vi "CC Script GUI.vi"(10 "Standalone":bool=TRUE, 11 "Cmd Qs":T1) -> ()   [LabVIEW 2021]
uses:
  Subsystems/SS cluster Command Queues.ctl
  Subsystems/SS typedef Cmd Queue Reference.ctl
  Subsystems/SS typedef cluster Instrument Command Queue Data.ctl
  CC cluster Script Panel Defaults.ctl
  typedefs/CC Script Step.ctl
  typedefs/CC enum Script Action.ctl
  typedefs/CC cluster Exposure.ctl
  Detector/Detector Class/Detector enum Detector Integration Mode.ctl
  typedefs/CC cluster Object.ctl
  typedefs/CC cluster sidereal rate.ctl
  typedefs/CC cluster RA and DEC.ctl
  typedefs/cc cluster muRA muDEC.ctl
  Telescope/CC cluster Telescope Offsets.ctl
  typedefs/CC cluster Acquire Parameters.ctl
  Subsystems/SS cluster Script Status Queue.ctl
  typedefs/CC cluster Random Dithering.ctl
  typedefs/CC Dithering.ctl
  typedefs/CC cluster Offset Dithering.ctl
  typedefs/CC Dithering Offsets.ctl
  typedefs/CC cluster Observation Record.ctl
  Subsystems/SS cluster New Image Data.ctl
  hk-channel-class/HK Item/HK Item.lvclass
  Subsystems/SS cluster Data Queue type.ctl
  typedefs/CC cluster Observation.ctl
  Observation Queue/CC enum Observation Status.ctl
  typedefs/CC cluster Observation Dither Options.ctl
  typedefs/CC enum Dither Selection.ctl
  typedefs/CC cluster Script.ctl
  typedefs/CC cluster Script Status Data.ctl
  typedefs/CC cluster Pause Parameters.ctl
  Filter Wheel/FW cmd Q Move Parameters.ctl
  Logging/CC enum Current Values Action.ctl
  Focus/Focus cluster MoveFocus Command Parameters.ctl
  CC Rd Wr Script Action.ctl
  e34a80dd-ae96-40f3-85ec-da568b1fc0c6.vi
  fb980131-14b8-4ba4-a5ba-d8795c8df878.vi
  73e8f019-b90d-454d-a375-f578a22e9470.vi
  6180e3d0-9506-4a5f-afbf-da5a1e2ce68c.vi
  79eba822-2b6b-4a1a-8f0f-f154aabb2b36.vi
  hk-channel-class/HK Table/HK Table.lvclass
  <vilib>/Utility/Data Type/NI_Data Type.lvlib
panel:
  in  "Script Path":path
  in  "Pause Button":bool
  out "Running":bool
  in  "Close":bool
  in  "Stop Script":bool
  in  "New Script":bool
  in  "Edit Script":bool
  in  "Run Script":bool
  in  "Script":string(combo)
  in  "Script":i32(listbox)
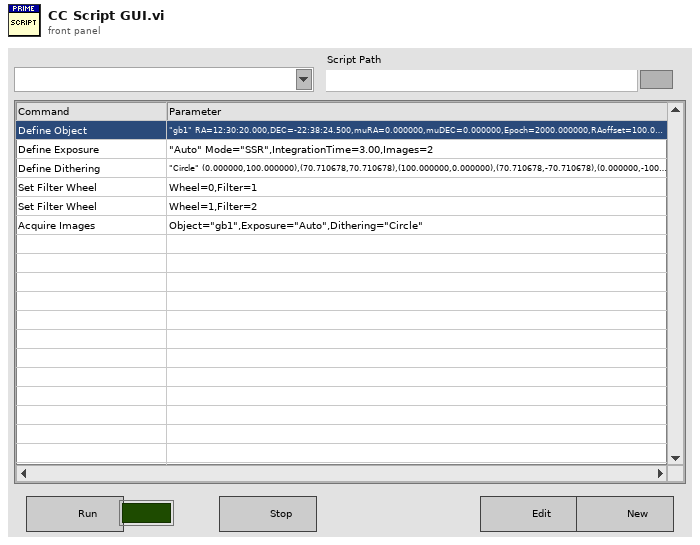
[diagram p1: front panel]
types:
  T1 = typedef "SS cluster Command Queues.ctl" = cluster{"Telescope Q":T2, "Filter Wheel Q":T2, "Script Q":T2, "CryoServer Q":T2, "Detector Q":T2, "Focus Q":T2}
  T2 = typedef "SS typedef Cmd Queue Reference.ctl" = refnum<queue>
  T3 = typedef "CC cluster Script Panel Defaults.ctl" = cluster{"Script Name":string, "Script Path":path}
  T4 = typedef "CC Script Step.ctl" = cluster{"Action":T5, "Data":variant}
  T5 = typedef "CC enum Script Action.ctl" = enum16{"Noop", "Define Object", "Define Exposure", "Define Dithering", "Acquire Images", "Set Filter Wheel", "Telescope Home", "Telescope Move", "Telescope RA DEC", "Focus Move Relative", "Focus Move Absolute", "Focus Set Home", "Macro", "Pause", "Ask User", "Define Random Dither"}
  T6 = typedef "CC cluster Exposure.ctl" = cluster{"Mode":T7, "Integration Time":dbl, "Name":string, "Images":i32}
  T7 = typedef "Detector enum Detector Integration Mode.ctl" = enum16{"SSR", "CDS", "MEAN", "MEDIAN", "MODE", "MIIN", "MAX"}
  T8 = typedef "CC cluster Object.ctl" = cluster{"Object":cluster{"Name":string}, "Sidereal Rate":T9, "RA and DEC":T10, "muRA muDEC Epoch":T11, "Offsets":T12}
  T9 = typedef "CC cluster sidereal rate.ctl" = cluster{"dRA":dbl, "dDEC":dbl}
  T10 = typedef "CC cluster RA and DEC.ctl" = cluster{"RA":dbl, "DEC":dbl}
  T11 = typedef "cc cluster muRA muDEC.ctl" = cluster{"muRA":dbl, "muDEC":dbl, "Epoch":dbl}
  T12 = typedef "CC cluster Telescope Offsets.ctl" = cluster{"RA":dbl, "DEC":dbl, "ROT":dbl}
  T13 = typedef "CC cluster Acquire Parameters.ctl" = cluster{"Object":string, "Exposure":string, "Dithering":string}
  T14 = typedef "CC cluster Random Dithering.ctl" = cluster{"Count":i32, "Radius":dbl, "Name":string}
  T15 = typedef "CC Dithering.ctl" = cluster{"Name":string, "Dithering Offsets":T16}
  T16 = typedef "CC cluster Offset Dithering.ctl" = cluster{"Offsets":T17[]}
  T17 = typedef "CC Dithering Offsets.ctl" = cluster{"DEC":dbl, "RA":dbl}
  T18 = typedef "CC cluster Observation Record.ctl" = cluster{"Start Time":timestamp, "Script":string, "Object":string, "Detector Settings":string, "Dithering Type":string, "Filter":string, "Images":i32}
  T19 = typedef "SS cluster New Image Data.ctl" = cluster{"Frame number":i32, "Detector #":u16, "FITS file":path, "File size":i64}
  T20 = typedef "CC cluster Observation.ctl" = cluster{"Priority":i32, "ID":string, "Observer":string, "Obj Name":string, "Obj Type":string, "RA and DEC String":cluster{"RA":string, "DEC":string}, "Filter Wheel 1":string, "Filter Wheel 2":string, "Integration Time":dbl, "Observation Status":T21, "Offsets":T12, "Images":i32, "Dither Options":T22, "Comment 1":string, "Comment 2":string}
  T21 = typedef "CC enum Observation Status.ctl" = enum16{"Ready", "Running", "Done", "Error"}
  T22 = typedef "CC cluster Observation Dither Options.ctl" = cluster{"Dither":T23, "Dither Radius":dbl, "Dither Points":i32, "Dither Phase":dbl}
  T23 = typedef "CC enum Dither Selection.ctl" = enum16{"None", "Circle", "Random"}
  T24 = cluster{"state":refnum<user-event>, "Script Settings":T3, "Script":T4[], "Cmd Qs":T1, "Parameters":variant, "step":i32, "Script Running":bool, "timer":timestamp, "Script State":string, "Exposure":T6, "Object Map":map{string, T8}, "Acq Settings":T13, "target":T8, "Exp Map":map{string, T6}, "Script Status Q":refnum<queue>, "Images Received":bool, "script edit ref":refnum<vi>, "Run Script":T4[], "Dither":cluster{"Dither Type":bool, "Random Dither":T14, "Offset Dithering":T15, "index":i32}, "Obs List":T18[], "Obs":T18, "images":T19[], "Channel List":refnum<class "HK Item.lvclass">[], "Data Q":refnum<queue>, "Total Images":i32, "paused":bool, "Target RA and DEC":T10, "Image idx":i32, "Observation":T20}
  T25 = enum8{"Enabled", "Disabled", "Disabled and Grayed Out"}
  T26 = typedef "SS typedef cluster Instrument Command Queue Data.ctl" = cluster{"Cmd":string, "Parameters":variant}
  T27 = typedef "SS cluster Data Queue type.ctl" = cluster{"Source":string, "Type":string, "Data":variant}
  T28 = typedef "SS cluster Script Status Queue.ctl" = cluster{"Msg":string, "Data":variant}
  T29 = typedef "CC cluster Script.ctl" = cluster{"Name":string, "Script":T4[]}
  T30 = typedef "CC cluster Script Status Data.ctl" = cluster{"Time":timestamp, "Running":bool, "Step":i32, "Script Name":string, "Step Name":string}
  T31 = typedef "CC cluster Pause Parameters.ctl" = cluster{"Time (s)":dbl}
  T32 = typedef "FW cmd Q Move Parameters.ctl" = cluster{"Wheel ID":i32, "Position":i32}
  T33 = typedef "CC enum Current Values Action.ctl" = enum16{"Init", "Write Item", "Write Array", "Read Item", "Read Array", "Read All", "Add Channels", "New File", "Add Message", "Get Current Values", "Close"}
  T34 = typedef "Focus cluster MoveFocus Command Parameters.ctl" = cluster{"Motor":i32, "Position":i32}
  T35 = typedef "CC Rd Wr Script Action.ctl" = enum16{"Read", "Write", "List", "Delete"}
  T36 = cluster{"Dither Type":bool, "Random Dither":T14, "Offset Dithering":T15, "index":i32}
  T37 = typedef "CC cluster Dithering.ctl" = cluster{"Dither Type":bool, "Random Dither":T14, "Offset Dithering":T15, "index":i32}
  T38 = typedef "LVPoint32TypeDef.ctl" = cluster{"Horizontal":i32, "Vertical":i32}
  T39 = typedef "LVRowAndColumnTypeDef.ctl" = cluster{"Row":i32, "Column":i32}
  T40 = enum32{"Invalid", "Standard", "Closed", "Hidden", "Minimized", "Maximized"}
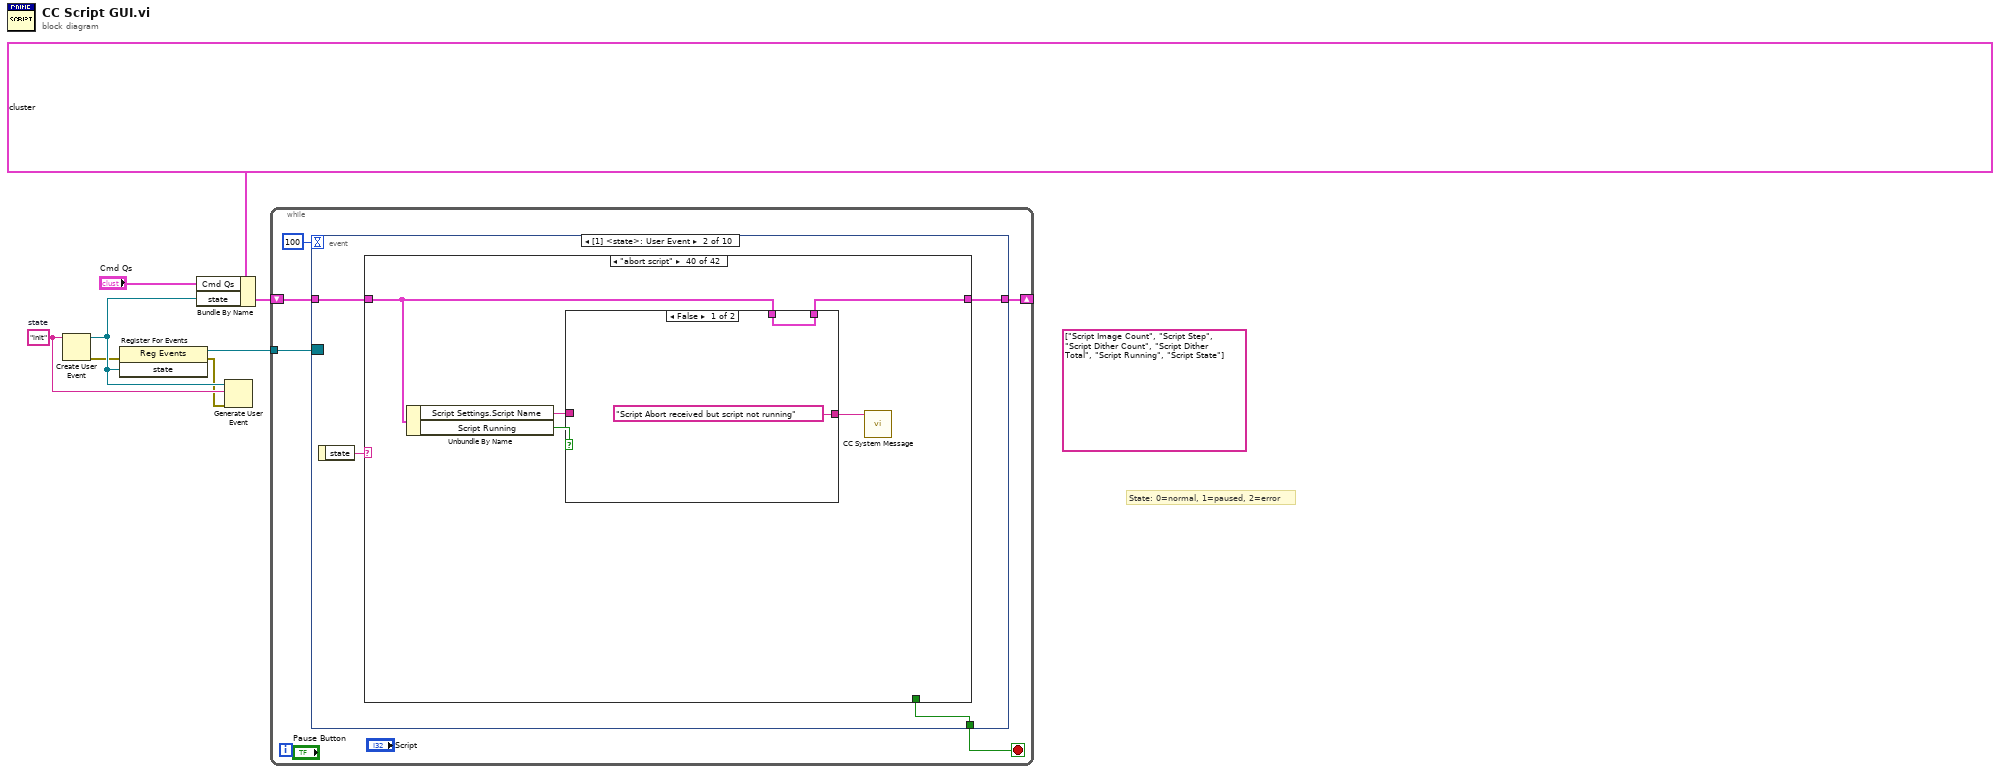
[diagram p0: block diagram]
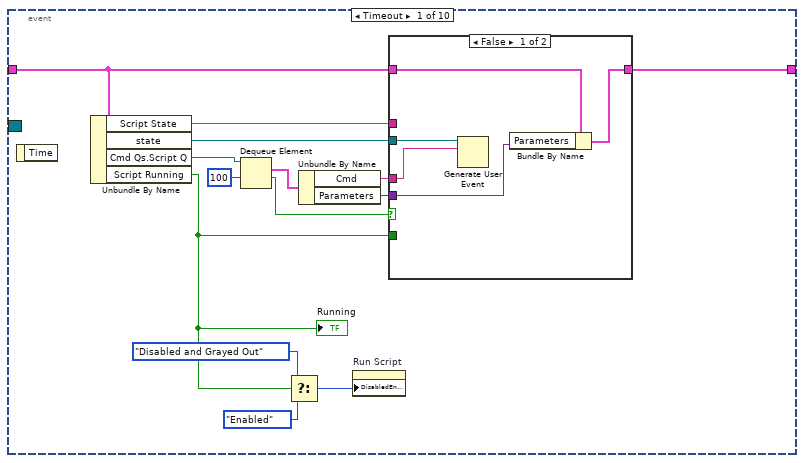
[diagram p2: hidden frame]
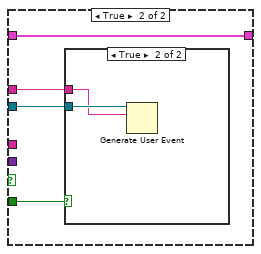
[diagram p3: hidden frame]
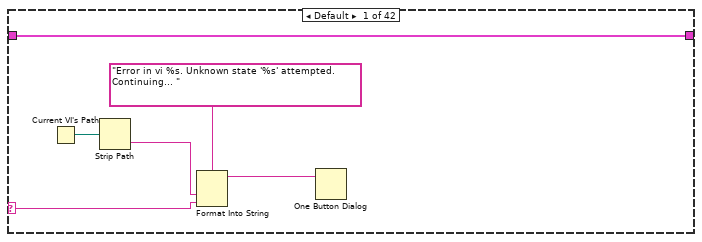
[diagram p5: hidden frame]
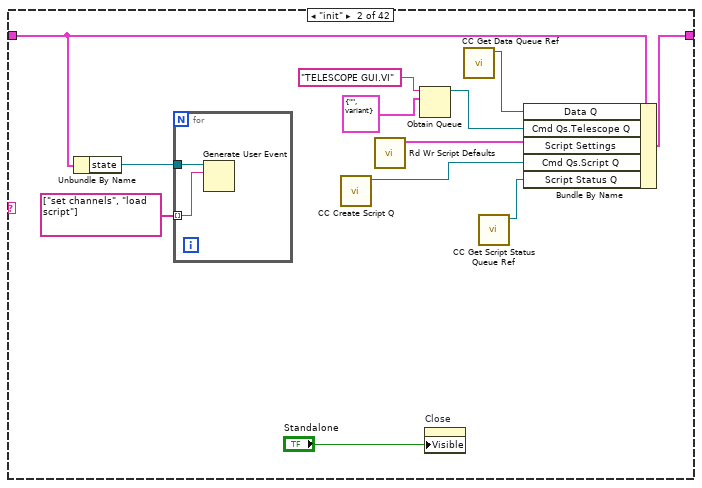
[diagram p6: hidden frame]
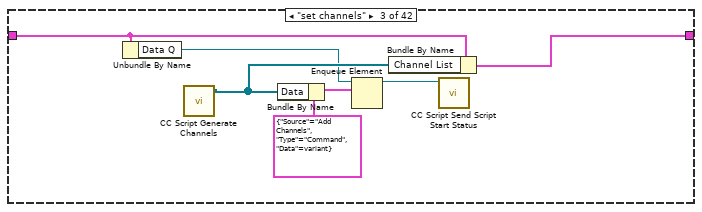
[diagram p7: hidden frame]
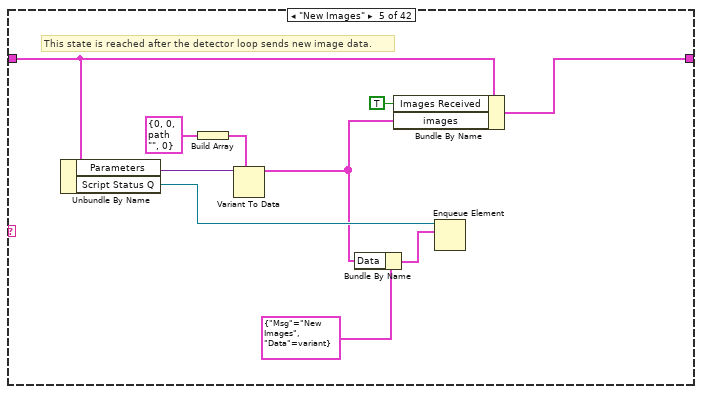
[diagram p9: hidden frame]
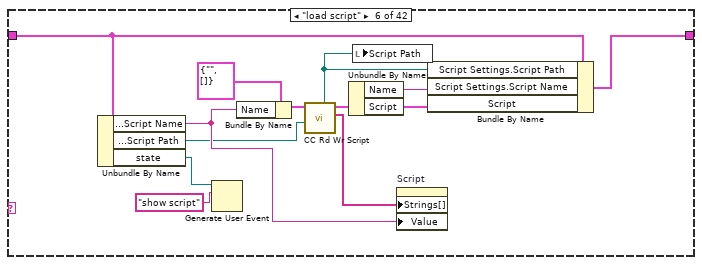
[diagram p10: hidden frame]
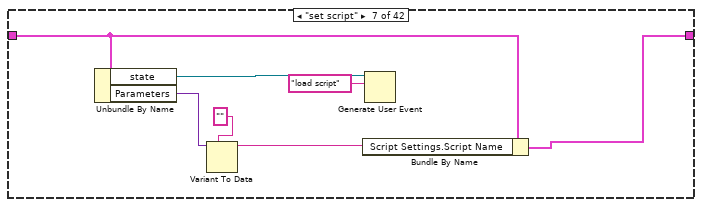
[diagram p11: hidden frame]
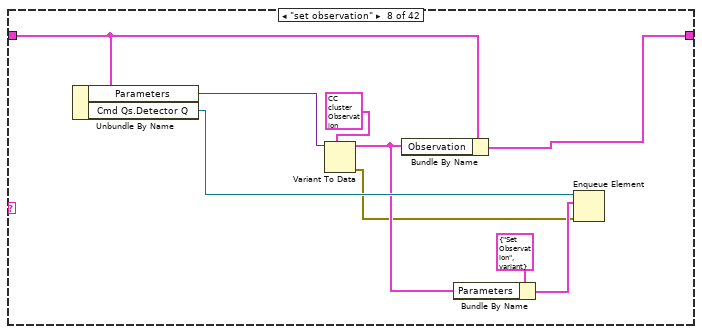
[diagram p12: hidden frame]
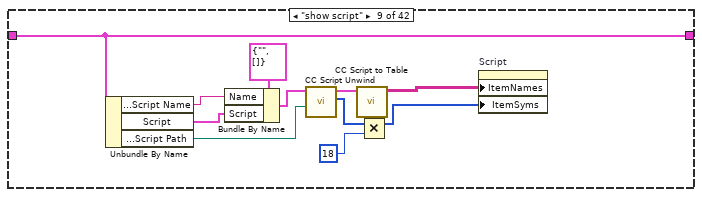
[diagram p13: hidden frame]
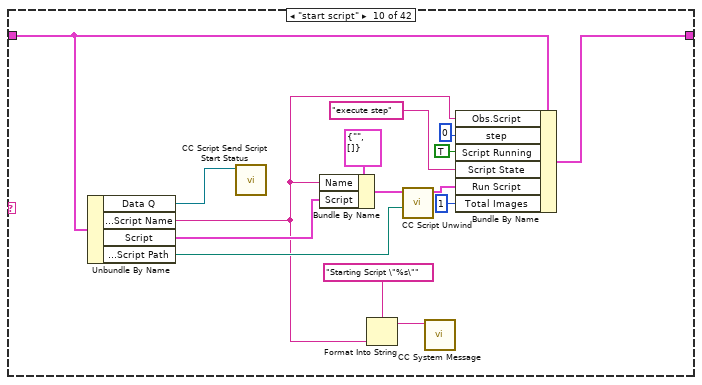
[diagram p14: hidden frame]
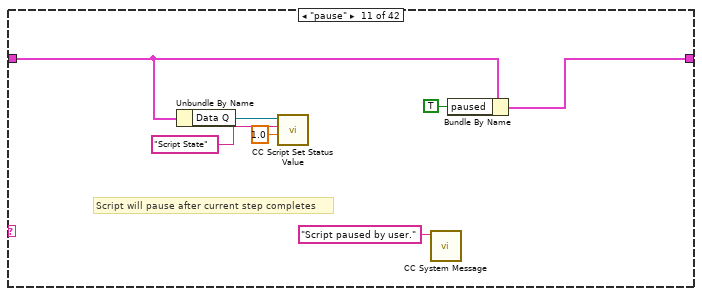
[diagram p15: hidden frame]
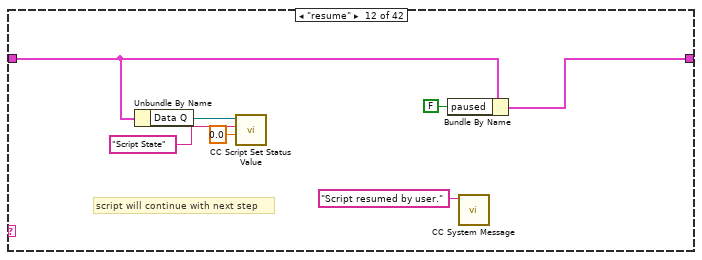
[diagram p16: hidden frame]
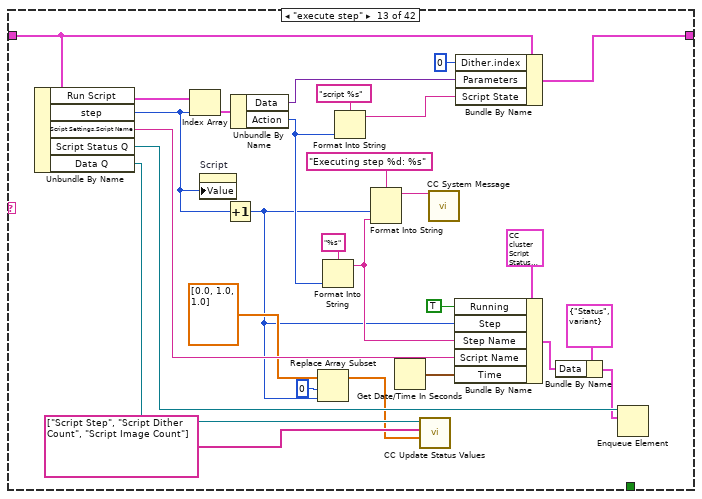
[diagram p17: hidden frame]
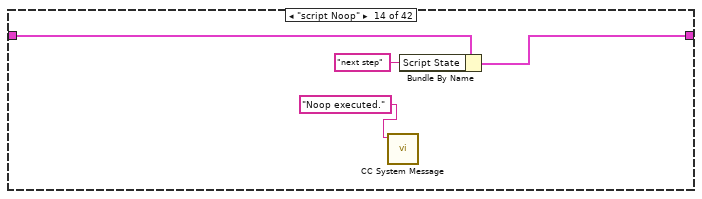
[diagram p18: hidden frame]
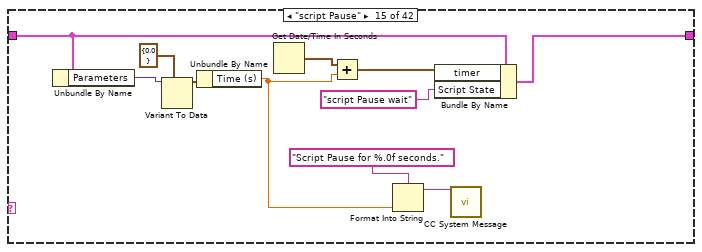
[diagram p19: hidden frame]
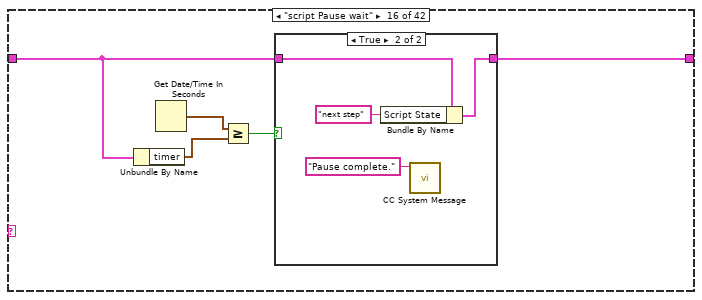
[diagram p20: hidden frame]
diagram:
  (unwired) string[] ["Script Image Count", "Script Step", "Script Dither Count", "Script Dither Total", "Script Running", "Script State"]
  w4 = "init"  # state
  # "State: 0=normal, 1=paused, 2=error"
  n1 = Create User Event(user event datatype=w4) -> (user event=w6:refnum<user-event>, error out=w2:errorcluster)  [unwired: 1 in]
  n2 = register-events(error in=w2, w6) -> (reference out=w5:refnum<event-registration>, error out=w3:errorcluster)  [unwired: 1 in]
  n3 = Bundle By Name(cluster=T24 {"state"=refnum, "Script Settings"={"Script Name"="", "Script Path"=path ""}, "Script"=[], "Cmd Qs"={"Telescope Q"=refnum, "Filter Wheel Q"=refnum, "Script Q"=refnum, "CryoServer Q"=refnum, "Detector Q"=refnum, "Focus Q"=refnum}, "Parameters"=variant, "step"=0, "Script Running"=FALSE, "timer"=timestamp(0 s since 1904-01-01), "Script State"="", "Exposure"={"Mode"=enum."CDS", "Integration Time"=1.0, "Name"="", "Images"=1}, "Object Map"={}, "Acq Settings"={"Object"="", "Exposure"="", "Dithering"=""}, "target"={"Object"={"Name"=""}, "Sidereal Rate"={"dRA"=0.0, "dDEC"=0.0}, "RA and DEC"={"RA"=0.0, "DEC"=0.0}, "muRA muDEC Epoch"={"muRA"=0.0, "muDEC"=0.0, "Epoch"=0.0}, "Offsets"={"RA"=0.0, "DEC"=0.0, "ROT"=0.0}}, "Exp Map"={}, "Script Status Q"=refnum, "Images Received"=FALSE, "script edit ref"=refnum, "Run Script"=[], "Dither"={"Dither Type"=FALSE, "Random Dither"={"Count"=1, "Radius"=1.0, "Name"=""}, "Offset Dithering"={"Name"="", "Dithering Offsets"={"Offsets"=[]}}, "index"=0}, "Obs List"=[], "Obs"={"Start Time"=timestamp(0 s since 1904-01-01), "Script"="", "Object"="", "Detector Settings"="", "Dithering Type"="", "Filter"="", "Images"=0}, "images"=[], "Channel List"=[], "Data Q"=refnum, "Total Images"=0, "paused"=FALSE, "Target RA and DEC"={"RA"=0.0, "DEC"=0.0}, "Image idx"=0, "Observation"={"Priority"=0, "ID"="", "Observer"="", "Obj Name"="", "Obj Type"="", "RA and DEC String"={"RA"="HH:MM:SS.nnn", "DEC"="DEG:arcmin:arcsec.nn"}, "Filter Wheel 1"="", "Filter Wheel 2"="", "Integration Time"=0.0, "Observation Status"=enum."Ready", "Offsets"={"RA"=0.0, "DEC"=0.0, "ROT"=0.0}, "Images"=0, "Dither Options"={"Dither"=enum."None", "Dither Radius"=0.0, "Dither Points"=0, "Dither Phase"=0.0}, "Comment 1"="", "Comment 2"=""}}, "Cmd Qs"="Cmd Qs", "state"=w6) -> (w7:T24)
  n4 = Generate User Event(user event=w6, event data cluster=w4, error in=w3) -> ()  [unwired: 1 in, 2 out]
  n5 = while {
    tunnel: w5 -> [w13]
    shift-right: [w11] -> _
    shift-left: w7 -> [w12]
    stop <- w10 stop-if-true
    n6 = event shown="[1] <state>: User Event" {
      selector: w13 -> [_ _ _ _ _ _ _ _ _ _]
      dyn-events: _ -> [_ _ _ _ _ _ _ _ _ _]
      timeout: 100 -> [_ _ _ _ _ _ _ _ _ _]
      tunnel: w12 -> [w21 w41 w654 w657 w672 w714 w719 w741 w744 w747]
      tunnel: [w19 w40 w651 w657 w671 w715 w720 w741 w744 w747] -> w11
      tunnel: [_ w39 _ _ _ _ _ _ _ _] -> w10
      event Timeout {
        n7 = event-data() -> ()  [unwired: 1 in, 1 out]
        n8 = Unbundle By Name(w21) -> ("Script State"=w18:string, "state"=w22:refnum<user-event>, "Cmd Qs.Script Q"=w27:T2, "Script Running"=w17:bool)
        "Running" <- w17
        n9 = Dequeue Element(queue=w27, timeout in ms (-1)=100) -> (element=w25:T26, timed out?=w24:bool)  [unwired: 1 in, 2 out]
        n10 = Select(t=T25."Disabled and Grayed Out" ("Disabled"), s=w17, f=T25."Enabled" ("Disabled")) -> (s? t:f=w14:T25)
        n11 = Unbundle By Name(w25) -> ("Cmd"=w23:string, "Parameters"=w20:variant)
        n12 = property on="Run Script" class="Bool"("DisabledEnum"=w14) -> ()  [unwired: 2 in, 2 out]
        n13 = case shown="False" w24 {
          tunnel: w23 -> [w31 _]
          tunnel: w22 -> [w32 w34]
          tunnel: w21 -> [w30 w36]
          tunnel: w20 -> [w29 _]
          tunnel: [w28 w36] -> w19
          tunnel: w17 -> [_ w35]
          tunnel: w18 -> [_ w33]
          frame False {
            n14 = Generate User Event(user event=w32, event data cluster=w31) -> ()  [unwired: 2 in, 2 out]
            n15 = Bundle By Name(cluster=w30, "Parameters"=w29) -> (w28:T24)
          }
          frame True {
            n16 = case shown="True" w35 {
              tunnel: w34 -> [_ w38]
              tunnel: w33 -> [_ w37]
              frame False {
              }
              frame True {
                n17 = Generate User Event(user event=w38, event data cluster=w37) -> ()  [unwired: 2 in, 2 out]
              }
            }
          }
        }
      }
      event User Event {
        n18 = event-data() -> ("state"=w42:string)  [unwired: 1 in]
        n19 = case shown="\"abort script\"" w42 {
          selector: w42 -> [w47 _ _ _ _ _ _ _ _ _ _ _ _ _ _ _ _ _ _ _ _ _ w291 _ _ _ _ _ _ w442 _ _ _ _ _ _ _ _ _ _ _ _]
          tunnel: w41 -> [w43 w58 w65 w70 w75 w84 w95 w107 w120 w134 w137 w147 w169 w178 w183 w194 w207 w228 w240 w255 w270 w287 w293 w314 w324 w334 w356 w381 w428 w439 w471 w496 w520 w533 w552 w561 w576 w592 w620 w628 w639 w647]
          tunnel: [w43 w59 w66 w70 w76 w85 w96 w108 w120 w135 w141 w148 w170 w179 w184 w193 w210 w229 w243 w258 w273 w289 w294 w316 w326 w336 w357 w384 w429 w440 w473 w494 w521 w534 w553 w562 w577 w590 w621 w629 w643 w647] -> w40
          tunnel: [_ _ _ _ _ _ _ _ _ _ _ _ _ _ _ _ _ _ _ _ _ _ _ _ _ _ _ _ _ _ _ _ _ _ _ _ _ _ _ _ _ TRUE] -> w39
          frame Default {
            n20 = Current VI's Path() -> (path=w46:path)
            n21 = Strip Path(path=w46) -> (name=w45:string)  [unwired: 1 out]
            n22 = Format Into String(format string="Error in vi %s. Unknown state '%s' attempted. Continuing... ", w45, w47) -> (resulting string=w44:string)  [unwired: 2 in, 1 out]
            n23 = One Button Dialog(message=w44) -> ()  [unwired: 1 in, 1 out]
          }
          frame "init" {
            n24 = Unbundle By Name(w58) -> ("state"=w57:refnum<user-event>)
            n25 = for {
              tunnel: w57 -> [w62]
              tunnel: string[] ["set channels", "load script"] -> [w61] mode=indexing
              n26 = Generate User Event(user event=w62, event data cluster=w61) -> ()  [unwired: 2 in, 2 out]
            }
            n27 = call "CC Create Script Q.vi"() -> ("Script Q"=w49:refnum<queue>)  [unwired: 10 in, 1 out]
            n28 = call "Rd Wr Script Defaults.vi"() -> ("Script Settings"=w60:T3)  [unwired: 10 in, 1 out]
            n29 = Obtain Queue(name (unnamed)="TELESCOPE GUI.VI", element data type=T26 {"Cmd"="", "Parameters"=variant}) -> (queue out=w52:refnum<queue>)  [unwired: 3 in, 2 out]
            n30 = property on="Close" class="Bool"("Visible"="Standalone") -> ()  [unwired: 2 in, 2 out]
            n31 = call "CC Get Data Queue Ref.vi"() -> ("Data Q"=w50:refnum<queue>)  [unwired: 10 in, 1 out]
            n32 = call "CC Get Script Status Queue Ref.vi"() -> ("Script Status Q"=w55:refnum<queue>)  [unwired: 10 in, 1 out]
            n33 = Bundle By Name(cluster=w58, "Data Q"=w50, "Cmd Qs.Telescope Q"=w52, "Script Settings"=w60, "Cmd Qs.Script Q"=w49, "Script Status Q"=w55) -> (w59:T24)
          }
          frame "set channels" {
            n34 = Unbundle By Name(w65) -> ("Data Q"=w64:refnum<queue>)
            n35 = call "CC Script Generate Channels.vi"() -> ("Channel List"=w67:refnum<class "HK Item.lvclass">[])  [unwired: 9 in, 2 out]
            n36 = Bundle By Name(cluster=T27 {"Source"="Add Channels", "Type"="Command", "Data"=variant} ("element"), "Data"=w67) -> (w69:T27)
            n37 = Enqueue Element(queue=w64, element=w69) -> (queue out=w63:refnum<queue>)  [unwired: 2 in, 2 out]
            n38 = Bundle By Name(cluster=w65, "Channel List"=w67) -> (w66:T24)
            n39 = call "CC Script Send Script Start Status.vi"("Data Q"=w63) -> ()  [unwired: 10 in, 1 out]
          }
          frame "idle" {
          }
          frame "New Images" {
            # "This state is reached after the detector loop sends new image data."
            n40 = Unbundle By Name(w75) -> ("Parameters"=w79:variant, "Script Status Q"=w74:refnum<queue>)
            n41 = Build Array(T19 {"Frame number"=0, "Detector #"=0, "FITS file"=path "", "File size"=0} ("New Image")) -> (w78:T19[])
            n42 = Variant To Data(type=w78, Variant=w79) -> (data=w71:T19[])  [unwired: 1 in, 1 out]
            n43 = Bundle By Name(cluster=T28 {"Msg"="New Images", "Data"=variant} ("element"), "Data"=w71) -> (w72:T28)
            n44 = Bundle By Name(cluster=w75, "Images Received"=TRUE, "images"=w71) -> (w76:T24)
            n45 = Enqueue Element(queue=w74, element=w72) -> ()  [unwired: 2 in, 3 out]
          }
          frame "load script" {
            n46 = Unbundle By Name(w84) -> ("Script Settings.Script Name"=w83:string, "Script Settings.Script Path"=w82:path, "state"=w88:refnum<user-event>)
            n47 = Generate User Event(user event=w88, event data cluster="show script" ("event data")) -> ()  [unwired: 2 in, 2 out]
            n48 = Bundle By Name(cluster=T29 {"Name"="", "Script"=[]} ("Script"), "Name"=w83) -> (w93:T29)
            n49 = call "CC Rd Wr Script.vi"("Script Path"=w82, "Script"=w93) -> ("Script List"=w91:string[], "Script"=w92:T29, "Script Path"=w81:path)  [unwired: 4 in, 3 out]
            n50 = Unbundle By Name(w92) -> ("Name"=w86:string, "Script"=w87:T4[])
            n51 = local write "Script Path"(w81) -> ()
            n52 = property on="Script" class="CmbBox"("Strings[]"=w91, "Value"=w83) -> ()  [unwired: 2 in, 2 out]
            n53 = Bundle By Name(cluster=w84, "Script Settings.Script Path"=w81, "Script Settings.Script Name"=w86, "Script"=w87) -> (w85:T24)
          }
          frame "set script" {
            n54 = Unbundle By Name(w95) -> ("state"=w98:refnum<user-event>, "Parameters"=w100:variant)
            n55 = Variant To Data(type="", Variant=w100) -> (data=w97:string)  [unwired: 1 in, 1 out]
            n56 = Bundle By Name(cluster=w95, "Script Settings.Script Name"=w97) -> (w96:T24)
            n57 = Generate User Event(user event=w98, event data cluster="load script" ("event data")) -> ()  [unwired: 2 in, 2 out]
          }
          frame "set observation" {
            n58 = Unbundle By Name(w107) -> ("Parameters"=w109:variant, "Cmd Qs.Detector Q"=w105:T2)
            n59 = Variant To Data(type=T20 {"Priority"=0, "ID"="", "Observer"="", "Obj Name"="", "Obj Type"="", "RA and DEC String"={"RA"="HH:MM:SS.nnn", "DEC"="DEG:arcmin:arcsec.nn"}, "Filter Wheel 1"="", "Filter Wheel 2"="", "Integration Time"=0.0, "Observation Status"=enum."Error", "Offsets"={"RA"=0.0, "DEC"=0.0, "ROT"=0.0}, "Images"=0, "Dither Options"={"Dither"=enum."None", "Dither Radius"=0.0, "Dither Points"=0, "Dither Phase"=0.0}, "Comment 1"="", "Comment 2"=""} ("element"), Variant=w109) -> (data=w102:T20, error out=w101:errorcluster)  [unwired: 1 in]
            n60 = Bundle By Name(cluster=w107, "Observation"=w102) -> (w108:T24)
            n61 = Bundle By Name(cluster=T26 {"Cmd"="Set Observation", "Parameters"=variant} ("element"), "Parameters"=w102) -> (w103:T26)
            n62 = Enqueue Element(queue=w105, element=w103, error in (no error)=w101) -> ()  [unwired: 1 in, 3 out]
          }
          frame "show script" {
            n63 = Unbundle By Name(w120) -> ("Script Settings.Script Name"=w117:string, "Script"=w116:T4[], "Script Settings.Script Path"=w110:path)
            n64 = Bundle By Name(cluster=T29 {"Name"="", "Script"=[]} ("Script"), "Name"=w117, "Script"=w116) -> (w115:T29)
            n65 = call "CC Script Unwind.vi"("Script Path"=w110, "Script"=w115) -> ("Indent"=w113:i32[], "Unwound Script"=w114:T4[])  [unwired: 7 in, 1 out]
            n66 = call "CC Script to Table.vi"("Script"=w114) -> ("table"=w119:string[][])  [unwired: 9 in, 1 out]
            n67 = Multiply(x=w113, y=18) -> (x*y=w112:i32[])
            n68 = property on="Script" class="MCListbox (strict)"("ItemNames"=w119, "ItemSyms"=w112) -> ()  [unwired: 2 in, 2 out]
          }
          frame "start script" {
            n69 = Unbundle By Name(w134) -> ("Data Q"=w122:refnum<queue>, "Script Settings.Script Name"=w123:string, "Script"=w127:T4[], "Script Settings.Script Path"=w124:path)
            n70 = call "CC Script Send Script Start Status.vi"("Data Q"=w122) -> ()  [unwired: 10 in, 1 out]
            n71 = Bundle By Name(cluster=T29 {"Name"="", "Script"=[]} ("Script"), "Name"=w123, "Script"=w127) -> (w126:T29)
            n72 = Format Into String(format string="Starting Script \"%s\"" ("Message"), w123) -> (resulting string=w131:string)  [unwired: 2 in, 1 out]
            n73 = call "CC Script Unwind.vi"("Script Path"=w124, "Script"=w126) -> ("Unwound Script"=w125:T4[])  [unwired: 7 in, 2 out]
            n74 = call "CC System Message.vi"("Message"=w131) -> ()  [unwired: 10 in, 1 out]
            n75 = Bundle By Name(cluster=w134, "Obs.Script"=w123, "step"=0, "Script Running"=TRUE, "Script State"="execute step" ("event data"), "Run Script"=w125, "Total Images"=1 ("Image Count")) -> (w135:T24)
          }
          frame "pause" {
            # "Script will pause after current step completes"
            n76 = Unbundle By Name(w137) -> ("Data Q"=w140:refnum<queue>)
            n77 = call "CC Script Set Status Value.vi"("Value"=1.0, "Ch Name"="Script State", "Data Q"=w140) -> ()  [unwired: 8 in, 1 out]
            n78 = call "CC System Message.vi"("Message"="Script paused by user.") -> ()  [unwired: 10 in, 1 out]
            n79 = Bundle By Name(cluster=w137, "paused"=TRUE) -> (w141:T24)
          }
          frame "resume" {
            # "script will continue with next step"
            n80 = Unbundle By Name(w147) -> ("Data Q"=w146:refnum<queue>)
            n81 = call "CC Script Set Status Value.vi"("Value"=0.0, "Ch Name"="Script State", "Data Q"=w146) -> ()  [unwired: 8 in, 1 out]
            n82 = Bundle By Name(cluster=w147, "paused"=FALSE) -> (w148:T24)
            n83 = call "CC System Message.vi"("Message"="Script resumed by user.") -> ()  [unwired: 10 in, 1 out]
          }
          frame "execute step" {
            n84 = Unbundle By Name(w169) -> ("Run Script"=w177:T4[], "step"=w173:i32, "Script Settings.Script Name"=w162:string, "Script Status Q"=w160:refnum<queue>, "Data Q"=w155:refnum<queue>)
            n85 = Index Array(array=w177, index=w173) -> (element=w176:T4)
            n86 = property on="Script" class="MCListbox (strict)"("Value"=w173) -> ()  [unwired: 2 in, 2 out]
            n87 = Increment(x=w173) -> (x+1=w151:i32)
            n88 = Unbundle By Name(w176) -> ("Data"=w168:variant, "Action"=w164:T5)
            n89 = Replace Array Subset(array=dbl[] [0.0, 1.0, 1.0] ("Values"), new element=w151, index=0) -> (w150:dbl[])
            n90 = Format Into String(format string="%s", w164) -> (resulting string=w163:string)  [unwired: 2 in, 1 out]
            n91 = Format Into String(format string="script %s", w164) -> (resulting string=w171:string)  [unwired: 2 in, 1 out]
            n92 = Format Into String(format string="Executing step %d: %s", w151, w163) -> (resulting string=w172:string)  [unwired: 2 in, 1 out]
            n93 = Get Date/Time In Seconds() -> (seconds since 1Jan1904=w161:timestamp)
            n94 = call "CC Update Status Values.vi"("Values"=w150, "names"=string[] ["Script Step", "Script Dither Count", "Script Image Count"], "Data Q"=w155) -> ()  [unwired: 8 in, 1 out]
            n95 = call "CC System Message.vi"("Message"=w172) -> ()  [unwired: 10 in, 1 out]
            n96 = Bundle By Name(cluster=T30 {"Time"=timestamp(0 s since 1904-01-01), "Running"=FALSE, "Step"=0, "Script Name"="", "Step Name"=""}, "Running"=TRUE, "Step"=w151, "Step Name"=w163, "Script Name"=w162, "Time"=w161) -> (w158:T30)
            n97 = Bundle By Name(cluster=w169, "Dither.index"=0, "Parameters"=w168, "Script State"=w171) -> (w170:T24)
            n98 = Bundle By Name(cluster=T28 {"Msg"="Status", "Data"=variant} ("element"), "Data"=w158) -> (w157:T28)
            n99 = Enqueue Element(queue=w160, element=w157) -> ()  [unwired: 2 in, 3 out]
          }
          frame "script Noop" {
            n100 = call "CC System Message.vi"("Message"="Noop executed." ("format string")) -> ()  [unwired: 10 in, 1 out]
            n101 = Bundle By Name(cluster=w178, "Script State"="next step" ("event data")) -> (w179:T24)
          }
          frame "script Pause" {
            n102 = Unbundle By Name(w183) -> ("Parameters"=w190:variant)
            n103 = Variant To Data(type=T31 {"Time (s)"=0.0} ("Pause Parameters"), Variant=w190) -> (data=w188:T31)  [unwired: 1 in, 1 out]
            n104 = Unbundle By Name(w188) -> ("Time (s)"=w186:dbl)
            n105 = Get Date/Time In Seconds() -> (seconds since 1Jan1904=w187:timestamp)
            n106 = Add(x=w187, y=w186) -> (x+y=w185:timestamp)
            n107 = Format Into String(format string="Script Pause for %.0f seconds.", w186) -> (resulting string=w191:string)  [unwired: 2 in, 1 out]
            n108 = Bundle By Name(cluster=w183, "timer"=w185, "Script State"="script Pause wait" ("event data")) -> (w184:T24)
            n109 = call "CC System Message.vi"("Message"=w191) -> ()  [unwired: 10 in, 1 out]
          }
          frame "script Pause wait" {
            n110 = Unbundle By Name(w194) -> ("timer"=w196:timestamp)
            n111 = Get Date/Time In Seconds() -> (seconds since 1Jan1904=w197:timestamp)
            n112 = Greater Or Equal?(x=w197, y=w196) -> (x >= y?=w195:bool)
            n113 = case shown="True" w195 {
              tunnel: w194 -> [w198 w202]
              tunnel: [w198 w200] -> w193
              frame False {
              }
              frame True {
                n114 = Bundle By Name(cluster=w202, "Script State"="next step") -> (w200:T24)
                n115 = call "CC System Message.vi"("Message"="Pause complete.") -> ()  [unwired: 10 in, 1 out]
              }
            }
          }
          frame "script Macro" {
            n116 = Unbundle By Name(w207) -> ("Parameters"=w208:variant)
            n117 = Variant To Data(type="", Variant=w208) -> (data=w204:string)  [unwired: 1 in, 1 out]
            n118 = Format Into String(format string="Executing Macro %s" ("Message"), w204) -> (resulting string=w203:string)  [unwired: 2 in, 1 out]
            n119 = Bundle By Name(cluster=w207, "Script State"="next step") -> (w210:T24)
            n120 = call "CC System Message.vi"("Message"=w203) -> ()  [unwired: 10 in, 1 out]
          }
          frame "script Define Object" {
            # "Move telescope"
            n121 = Unbundle By Name(w228) -> ("Parameters"=w227:variant, "Object Map"=w225:map{string, T8}, "Cmd Qs.Telescope Q"=w212:T2)
            n122 = Variant To Data(type=T8 {"Object"={"Name"=""}, "Sidereal Rate"={"dRA"=0.0, "dDEC"=0.0}, "RA and DEC"={"RA"=0.0, "DEC"=0.0}, "muRA muDEC Epoch"={"muRA"=0.0, "muDEC"=0.0, "Epoch"=0.0}, "Offsets"={"RA"=0.0, "DEC"=0.0, "ROT"=0.0}} ("Object"), Variant=w227) -> (data=w211:T8)  [unwired: 1 in, 1 out]
            n123 = Unbundle By Name(w211) -> ("Object.Name"=w224:string)
            n124 = Unbundle By Name(w211) -> ("Object.Name"=w221:string, "RA and DEC.RA"=w220:dbl, "RA and DEC.DEC"=w219:dbl, "Offsets.RA"=w217:dbl, "Offsets.DEC"=w216:dbl, "Offsets.ROT"=w215:dbl)
            n125 = Insert Into Map(map in=w225, key=w224, value=w211) -> (map out=w223:map{string, T8})  [unwired: 2 out]
            n126 = Bundle By Name(cluster=w228, "Script State"="next step", "Object Map"=w223) -> (w229:T24)
            n127 = Bundle By Name(cluster=T26 {"Cmd"="Move", "Parameters"=variant} ("element"), "Parameters"=w211) -> (w213:T26)
            n128 = Format Into String(format string="Script defined target object \"%s\" at RA=%f, DEC=%f and RAoffset=%.1f, DECoffset=%.1f, ROToffset=%.1g", w221, w220, w219, w217, w216, w215) -> (resulting string=w218:string)  [unwired: 2 in, 1 out]
            n129 = Enqueue Element(queue=w212, element=w213) -> ()  [unwired: 2 in, 3 out]
            n130 = call "CC System Message.vi"("Message"=w218) -> ()  [unwired: 10 in, 1 out]
          }
          frame "script Define Exposure" {
            n131 = Unbundle By Name(w240) -> ("Exp Map"=w239:map{string, T6}, "Parameters"=w242:variant)
            n132 = Variant To Data(type=T6 {"Mode"=enum."CDS", "Integration Time"=1.0, "Name"="", "Images"=1} ("Exposure"), Variant=w242) -> (data=w237:T6)  [unwired: 1 in, 1 out]
            n133 = Unbundle By Name(w237) -> ("Images"=w231:i32, "Name"=w234:string, "Mode"=w233:T7, "Integration Time"=w232:dbl)
            n134 = Insert Into Map(map in=w239, key=w234, value=w237) -> (map out=w238:map{string, T6})  [unwired: 2 out]
            n135 = Bundle By Name(cluster=w240, "Script State"="next step", "Exp Map"=w238, "Image idx"=w231) -> (w243:T24)
            n136 = Format Into String(format string="Script defined exposure settings \"%s\" mode %s, integration time %f, collection %d images.", w234, w233, w232, w231) -> (resulting string=w235:string)  [unwired: 2 in, 1 out]
            n137 = call "CC System Message.vi"("Message"=w235) -> ()  [unwired: 10 in, 1 out]
          }
          frame "script Define Random Dither" {
            n138 = Unbundle By Name(w255) -> ("Parameters"=w257:variant, "Data Q"=w248:refnum<queue>)
            n139 = Variant To Data(type=T14 {"Count"=1, "Radius"=1.0, "Name"=""} ("Dithering Offsets"), Variant=w257) -> (data=w251:T14)  [unwired: 1 in, 1 out]
            n140 = Unbundle By Name(w251) -> ("Name"=w250:string, "Count"=w246:i32, "Radius"=w249:dbl)
            n141 = Increment(x=w246) -> (x+1=w245:i32)
            n142 = Bundle By Name(cluster=w255, "Script State"="next step", "Dither.Random Dither"=w251, "Dither.Dither Type"=TRUE) -> (w258:T24)
            n143 = Format Into String(format string="Script defined random dithering \"%s\" at %d spots with radius %f", w250, w246, w249) -> (resulting string=w252:string)  [unwired: 2 in, 1 out]
            n144 = call "CC Script Set Status Value.vi"("Value"=w245, "Ch Name"="Script Dither Total", "Data Q"=w248) -> ()  [unwired: 8 in, 1 out]
            n145 = call "CC System Message.vi"("Message"=w252) -> ()  [unwired: 10 in, 1 out]
          }
          frame "script Define Dithering" {
            n146 = Unbundle By Name(w270) -> ("Parameters"=w272:variant, "Data Q"=w262:refnum<queue>)
            n147 = Variant To Data(type=T15 {"Name"="", "Dithering Offsets"={"Offsets"=[]}} ("Dithering Offsets"), Variant=w272) -> (data=w266:T15)  [unwired: 1 in, 1 out]
            n148 = Unbundle By Name(w266) -> ("Name"=w265:string, "Dithering Offsets.Offsets"=w264:T17[])
            n149 = Bundle By Name(cluster=w270, "Script State"="next step", "Dither.Offset Dithering"=w266, "Dither.Dither Type"=FALSE) -> (w273:T24)
            n150 = Array Size(array=w264) -> (size(s)=w261:i32)
            n151 = Increment(x=w261) -> (x+1=w260:i32)
            n152 = Format Into String(format string="Script defined dithering \"%s\" containing %d offsets.", w265, w261) -> (resulting string=w267:string)  [unwired: 2 in, 1 out]
            n153 = call "CC Script Set Status Value.vi"("Value"=w260, "Ch Name"="Script Dither Total", "Data Q"=w262) -> ()  [unwired: 8 in, 1 out]
            n154 = call "CC System Message.vi"("Message"=w267) -> ()  [unwired: 10 in, 1 out]
          }
          frame "script Set Filter Wheel" {
            n155 = Unbundle By Name(w287) -> ("Parameters"=w288:variant, "Cmd Qs.Filter Wheel Q"=w286:T2)
            n156 = Variant To Data(type=T32 {"Wheel ID"=0, "Position"=0}, Variant=w288) -> (data=w277:T32, error out=w283:errorcluster)  [unwired: 1 in]
            n157 = Bundle By Name(cluster=T26 {"Cmd"="Move", "Parameters"=variant} ("element"), "Parameters"=w277) -> (w278:T26)
            n158 = Enqueue Element(queue=w286, element=w278, error in (no error)=w283) -> (error out=w282:errorcluster)  [unwired: 1 in, 2 out]
            n159 = Unbundle By Name(w277) -> ("Wheel ID"=w276:i32, "Position"=w275:i32)
            n160 = call "Stall Data Flow.vim"("value in"=w282, "milliseconds to wait"=u32 5000) -> ()  [unwired: 2 out]
            n161 = Format Into String(format string="Script moving filter wheel %d to position %d", w276, w275) -> (resulting string=w279:string)  [unwired: 2 in, 1 out]
            n162 = Bundle By Name(cluster=w287, "Script State"="script Filter Wheel Wait") -> (w289:T24)
            n163 = call "CC System Message.vi"("Message"=w279) -> ()  [unwired: 10 in, 1 out]
          }
          frame "script Filter Wheel Wait" {
            n164 = call "CC Log Object.vi"("Action"=CC_enum_Current_Values_Action."Get Current Values") -> ("HK Channel out"=w301:refnum<class "HK Table.lvclass">)  [unwired: 8 in, 2 out]
            n165 = for {
              N: 2 -> [_]
              tunnel: w301 -> [w307]
              tunnel: [w306] -> w298 mode=indexing
              tunnel: "Wheel%d Moving" -> [w305]
              i -> [w304]
              n166 = Format Into String(format string=w305, w304) -> (resulting string=w303:string)  [unwired: 2 in, 1 out]
              n167 = call-dynamic "HK Read Value.vi"("Channel Name"=w303, "HK Channel in"=w307) -> ("Value"=w306:dbl)  [unwired: 4 in, 5 out]
            }
            n168 = Equal To 0?(x=w298) -> (x = 0?=w297:bool[])
            n169 = And Array Elements(Boolean array=w297) -> (logical AND=w296:bool)
            n170 = Select(t="next step", s=w296, f=w291) -> (s? t:f=w295:string)
            n171 = Bundle By Name(cluster=w293, "Script State"=w295) -> (w294:T24)
          }
          frame "script Focus Move Relative" {
            n172 = Unbundle By Name(w314) -> ("Parameters"=w315:variant, "Cmd Qs.Focus Q"=w313:T2)
            n173 = Variant To Data(type=T34 {"Motor"=0, "Position"=0} ("Cluster"), Variant=w315) -> (data=w311:T34, error out=w310:errorcluster)  [unwired: 1 in]
            n174 = Bundle By Name(cluster=T26 {"Cmd"="FocusMoveRelative", "Parameters"=variant} ("element"), "Parameters"=w311) -> (w309:T26)
            n175 = Enqueue Element(queue=w313, element=w309, error in (no error)=w310) -> ()  [unwired: 1 in, 3 out]
            n176 = Bundle By Name(cluster=w314, "Script State"="next step") -> (w316:T24)
          }
          frame "script Focus Move Absolute" {
            n177 = Unbundle By Name(w324) -> ("Parameters"=w325:variant, "Cmd Qs.Focus Q"=w323:T2)
            n178 = Variant To Data(type=T34 {"Motor"=0, "Position"=0} ("Cluster"), Variant=w325) -> (data=w321:T34, error out=w320:errorcluster)  [unwired: 1 in]
            n179 = Bundle By Name(cluster=T26 {"Cmd"="FocusMoveAbsolute", "Parameters"=variant} ("element"), "Parameters"=w321) -> (w319:T26)
            n180 = Enqueue Element(queue=w323, element=w319, error in (no error)=w320) -> ()  [unwired: 1 in, 3 out]
            n181 = Bundle By Name(cluster=w324, "Script State"="next step") -> (w326:T24)
          }
          frame "script Focus Set Home" {
            n182 = Unbundle By Name(w334) -> ("Parameters"=w335:variant, "Cmd Qs.Focus Q"=w333:T2)
            n183 = Variant To Data(type=0, Variant=w335) -> (data=w331:i32, error out=w330:errorcluster)  [unwired: 1 in]
            n184 = Bundle By Name(cluster=T26 {"Cmd"="FocusSetHome", "Parameters"=variant} ("element"), "Parameters"=w331) -> (w329:T26)
            n185 = Enqueue Element(queue=w333, element=w329, error in (no error)=w330) -> ()  [unwired: 1 in, 3 out]
            n186 = Bundle By Name(cluster=w334, "Script State"="next step") -> (w336:T24)
          }
          frame "script Acquire Images" {
            # "Tell the telescope to move to target."
            n187 = Unbundle By Name(w356) -> ("Exp Map"=w340:map{string, T6}, "Object Map"=w355:map{string, T8}, "Parameters"=w360:variant, "Cmd Qs.Telescope Q"=w358:T2, "Data Q"=w346:refnum<queue>)
            n188 = Variant To Data(type=T13 {"Object"="", "Exposure"="", "Dithering"=""} ("Acquire Parameters"), Variant=w360) -> (data=w341:T13)  [unwired: 1 in, 1 out]
            n189 = Unbundle By Name(w341) -> ("Exposure"=w339:string)
            n190 = Unbundle By Name(w341) -> ("Object"=w347:string)
            n191 = call "CC Script Set Status Value.vi"("Value"=1.0, "Ch Name"="Script Dither Count", "Data Q"=w346) -> ()  [unwired: 8 in, 1 out]
            n192 = Remove From Map(10:w339, 11:w340) -> (1:w338:T6)  [unwired: 2 out]
            n193 = Remove From Map(10:w347, 11:w355) -> (1:w354:T8, 2:w353:bool)  [unwired: 1 out]
            n194 = case shown="False" w353 {
              tunnel: w358 -> [w363 _]
              tunnel: w354 -> [w361 w368]
              tunnel: ["script Acquire Wait Move" ("Script State") "abort script" ("Script State")] -> w352
              tunnel: w347 -> [_ w370]
              tunnel: [w361 w368] -> w343
              frame False {
                n195 = disable-structure shown="Enabled" {
                  disable-tunnel: w363 -> [w367 _]
                  disable-tunnel: w361 -> [w364 _]
                  frame Disabled {
                    n196 = Bundle By Name(cluster=T26 {"Cmd"="Move", "Parameters"=variant} ("element"), "Parameters"=w364) -> (w365:T26)
                    n197 = Enqueue Element(queue=w367, element=w365) -> ()  [unwired: 2 in, 3 out]
                  }
                  frame Enabled {
                    # "Telescope move command\nnow in the Define Object\nstep to save time."
                  }
                }
              }
              frame True {
                n198 = Format Into String(format string="Acquire Images command referred to undefined object \"%s\".", w370) -> (resulting string=w369:string)  [unwired: 2 in, 1 out]
                n199 = call "CC System Message.vi"("Message"=w369) -> ()  [unwired: 10 in, 1 out]
                n200 = One Button Dialog(message=w369) -> ()  [unwired: 1 in, 1 out]
              }
            }
            n201 = Unbundle By Name(w343) -> ("RA and DEC"=w342:T10)
            n202 = Format Into String(format string="Waiting for telescope to target %s", w347) -> (resulting string=w348:string)  [unwired: 2 in, 1 out]
            n203 = call "CC System Message.vi"("Message"=w348) -> ()  [unwired: 10 in, 1 out]
            n204 = Get Date/Time In Seconds() -> (seconds since 1Jan1904=w351:timestamp)
            n205 = Bundle By Name(cluster=w356, "Dither.index"=0, "Acq Settings"=w341, "timer"=w351, "Exposure"=w338, "target"=w343, "Target RA and DEC"=w342, "Script State"=w352) -> (w357:T24)
          }
          frame "script Acquire Wait Move" {
            # "Wait for telescope to finish moving."
            n206 = Unbundle By Name(w381) -> ("timer"=w376:timestamp, "Target RA and DEC"=w380:T10, "Exposure.Images"=w373:i32)
            n207 = call "CC Log Object.vi"("Action"=CC_enum_Current_Values_Action."Get Current Values") -> ("HK Channel out"=w388:refnum<class "HK Table.lvclass">)  [unwired: 8 in, 2 out]
            n208 = Get Date/Time In Seconds() -> (seconds since 1Jan1904=w378:timestamp)
            n209 = for {
              tunnel: w388 -> [w392]
              tunnel: string[] ["Telescope RA", "Telescope DEC", "Telescope Moving?", "Telescope Status"] -> [w391] mode=indexing
              tunnel: [w390] -> w386 mode=indexing
              n210 = call-dynamic "HK Read Value.vi"("Channel Name"=w391, "HK Channel in"=w392) -> ("Value"=w390:dbl)  [unwired: 4 in, 5 out]
            }
            n211 = Subtract(x=w378, y=w376) -> (x-y=w379:dbl)
            n212 = Less?(x=w379, y=180.0) -> (x < y?=w375:bool)
            n213 = Index Array(array=w386) -> (element #1=w383:dbl, element #2=w382:dbl, element #3=w385:dbl)  [unwired: 4 in, 1 out]
            n214 = Equal To 0?(x=w385) -> (x = 0?=w374:bool)
            n215 = case shown="True" w374 {
              tunnel: w381 -> [w393 w407]
              tunnel: [w394 w408] -> w384
              tunnel: w383 -> [_ w411]
              tunnel: w382 -> [_ w410]
              tunnel: w380 -> [_ w412]
              tunnel: w375 -> [w395 _]
              tunnel: w373 -> [_ w405]
              frame False {
                n216 = case shown="True" w395 {
                  tunnel: w393 -> [w398 w400]
                  tunnel: [w397 w400] -> w394
                  frame False {
                    n217 = call "CC System Message.vi"("Message"="Timeout waiting for telescope to reach position.") -> ()  [unwired: 10 in, 1 out]
                    n218 = Bundle By Name(cluster=w398, "Script State"="Script Error") -> (w397:T24)
                  }
                  frame True {
                  }
                }
              }
              frame True {
                # "Not moving"
                n219 = Bundle(cluster=w412, "RA"=w411, "DEC"=w410) -> (w409:T10)
                n220 = call "CC Script Check Telescope is Close Enough.vi"("Current Pos"=w409, "Target Pos"=w412) -> ("msg"=w401:string, "close enough"=w404:bool)  [unwired: 7 in, 1 out]
                n221 = case shown="True" w404 {
                  tunnel: w405 -> [_ w415]
                  tunnel: w401 -> [w413 _]
                  frame False {
                    n222 = call "CC System Message.vi"("Message"=w413) -> ()  [unwired: 10 in, 1 out]
                  }
                  frame True {
                    n223 = Format Into String(format string="Image 1 of %d.", w415) -> (resulting string=w414:string)  [unwired: 2 in, 1 out]
                    n224 = call "CC System Message.vi"("Message"=w414) -> ()  [unwired: 10 in, 1 out]
                  }
                }
                n225 = Select(t="script Read Detectors", s=w404, f="Script Error" ("Script State")) -> (s? t:f=w406:string)
                n226 = Bundle By Name(cluster=w407, "Script State"=w406) -> (w408:T24)
              }
            }
          }
          frame "script Read Detectors" {
            n227 = Unbundle By Name(w428) -> ("Exp Map"=w435:map{string, T6}, "Acq Settings.Exposure"=w434:string, "Cmd Qs.Detector Q"=w433:T2)
            n228 = Remove From Map(10:w434, 11:w435) -> (1:w419:T6)  [unwired: 2 out]
            n229 = Unbundle By Name(w419) -> ("Images"=w420:i32, "Name"=w423:string, "Mode"=w422:T7, "Integration Time"=w421:dbl)
            n230 = Bundle By Name(cluster=T26 {"Cmd"="Acquire Image", "Parameters"=variant} ("element"), "Parameters"=w419) -> (w431:T26)
            n231 = Enqueue Element(queue=w433, element=w431) -> ()  [unwired: 2 in, 3 out]
            n232 = Get Date/Time In Seconds() -> (seconds since 1Jan1904=w427:timestamp)
            n233 = Format Into String(format string="Detector exposure settings \"%s\" mode %s, integration time %f, collection %d images.", w423, w422, w421, w420) -> (resulting string=w417:string)  [unwired: 2 in, 1 out]
            n234 = Bundle By Name(cluster=w428, "timer"=w427, "Script State"="script Wait for Image", "Images Received"=FALSE) -> (w429:T24)
            n235 = call "CC System Message.vi"("Message"="Commanding Detetor to acquire images." ("format string")) -> ("error out"=w418:errorcluster)  [unwired: 10 in]
            n236 = call "CC System Message.vi"("error in (no error)"=w418, "Message"=w417) -> ()  [unwired: 9 in, 1 out]
          }
          frame "script Wait for Image" {
            # "Waiting for detector system to return images via script Q. State \"New Images\" sets the state so we can move on."
            n237 = Unbundle By Name(w439) -> ("timer"=w438:timestamp, "Images Received"=w443:bool, "Acq Settings"=w437:T13)
            n238 = Get Date/Time In Seconds() -> (seconds since 1Jan1904=w447:timestamp)
            n239 = Subtract(x=w447, y=w438) -> (x-y=w446:dbl)
            n240 = Greater?(x=w446, y=180.0) -> (0:w444:bool)
            n241 = case shown="False" w444 {
              tunnel: w443 -> [w457 _]
              tunnel: w442 -> [w456 _]
              tunnel: [w454 "Script Error"] -> w441
              tunnel: w439 -> [w453 w458]
              tunnel: w437 -> [w452 _]
              tunnel: [w448 w458] -> w436
              frame False {
                n242 = Unbundle By Name(w452) -> ("Object"=w451:string, "Exposure"=w450:string, "Dithering"=w449:string)
                n243 = Select(t="Next Image", s=w457, f=w456) -> (s? t:f=w454:string)
                n244 = Bundle By Name(cluster=w453, "Obs.Object"=w451, "Obs.Detector Settings"=w450, "Obs.Dithering Type"=w449) -> (w448:T24)
              }
              frame True {
                # "time out. Report error and abort"
                n245 = call "CC System Message.vi"("Message"="Timeout waiting for detector to return images.") -> ()  [unwired: 10 in, 1 out]
              }
            }
            n246 = Bundle By Name(cluster=w436, "Script State"=w441) -> (w440:T24)
          }
          frame "Next Image" {
            n247 = Unbundle By Name(w471) -> ("Exposure.Images"=w463:i32, "Image idx"=w468:i32, "Data Q"=w470:refnum<queue>, "Total Images"=w469:i32)
            n248 = Increment(x=w469) -> (x+1=w462:i32)
            n249 = Decrement(x=w468) -> (x-1=w466:i32)
            n250 = call "CC Script Set Status Value.vi"("Value"=w462, "Ch Name"="Script Image Count", "Data Q"=w470) -> ()  [unwired: 8 in, 1 out]
            n251 = Greater Than 0?(x=w466) -> (x > 0?=w467:bool)
            n252 = case shown="True" w467 {
              tunnel: w466 -> [_ w481]
              tunnel: [w475 w481] -> w465
              tunnel: ["Next Dither" "script Read Detectors"] -> w464
              tunnel: w463 -> [w475 w479]
              tunnel: ["Images complete. Going to next dither." w478] -> w461
              frame False {
              }
              frame True {
                n253 = Subtract(x=w479, y=w481) -> (x-y=w480:i32)
                n254 = Increment(x=w480) -> (x+1=w477:i32)
                n255 = Format Into String(format string="Image %d of %d.", w477, w479) -> (resulting string=w478:string)  [unwired: 2 in, 1 out]
              }
            }
            n256 = Bundle By Name(cluster=w471, "Image idx"=w465, "Script State"=w464, "Total Images"=w462) -> (w473:T24)
            n257 = call "CC System Message.vi"("Message"=w461) -> ()  [unwired: 10 in, 1 out]
          }
          frame "Next Dither" {
            n258 = Unbundle By Name(w496) -> ("Dither"=w492:T36, "target"=w491:T8, "Cmd Qs.Telescope Q"=w497:T2, "Data Q"=w488:refnum<queue>)
            n259 = call "CC Script Next Dither.vi"("object"=w491, "Dither"=w492) -> ("Dither?"=w490:bool, "object"=w486:T8, "Dither out"=w487:T37, "Message"=w484:string)  [unwired: 5 in, 1 out]
            n260 = case shown="True" w490 {
              tunnel: w486 -> [_ w514]
              tunnel: w497 -> [_ w513]
              tunnel: ["Next Step" "script Acquire Wait Move" ("Script State")] -> w495
              tunnel: ["Image acquisition and dithering complete." ("format string") w506] -> w489
              tunnel: w487 -> [_ w510]
              tunnel: w488 -> [w499 w508]
              tunnel: w484 -> [_ w506]
              frame False {
                w498 = 0.0 ("Value")
                n261 = call "CC Script Set Status Value.vi"("Value"=w498, "Ch Name"="Script Dither Total", "Data Q"=w499) -> ()  [unwired: 8 in, 1 out]
                n262 = call "CC Script Set Status Value.vi"("Value"=w498, "Ch Name"="Script Dither Count", "Data Q"=w499) -> ()  [unwired: 8 in, 1 out]
              }
              frame True {
                n263 = Bundle By Name(cluster=T26 {"Cmd"="Move", "Parameters"=variant} ("element"), "Parameters"=w514) -> (w516:T26)
                n264 = Unbundle By Name(w510) -> ("index"=w511:i32)
                n265 = Increment(x=w511) -> (x+1=w509:i32)
                n266 = call "CC Script Set Status Value.vi"("Value"=w509, "Ch Name"="Script Dither Count", "Data Q"=w508) -> ()  [unwired: 8 in, 1 out]
                n267 = Enqueue Element(queue=w513, element=w516) -> (error out=w505:errorcluster)  [unwired: 2 in, 2 out]
                n268 = call "Stall Data Flow.vim"("value in"=w505, "milliseconds to wait"=u32 4000) -> ()  [unwired: 2 out]
              }
            }
            n269 = Unbundle By Name(w486) -> ("RA and DEC"=w485:T10)
            n270 = Get Date/Time In Seconds() -> (seconds since 1Jan1904=w493:timestamp)
            n271 = Bundle By Name(cluster=w496, "timer"=w493, "Target RA and DEC"=w485, "Dither"=w487, "Script State"=w495) -> (w494:T24)
            n272 = call "CC System Message.vi"("Message"=w489) -> ()  [unwired: 10 in, 1 out]
          }
          frame "script Telescope Move" {
            # "give telescope time to start\nmoving."
            n273 = Unbundle By Name(w520) -> ("Run Script"=w529:T4[], "step"=w528:i32, "Cmd Qs.Telescope Q"=w526:T2)
            n274 = Index Array(array=w529, index=w528) -> (element=w527:T4)
            n275 = Unbundle By Name(w527) -> ("Data"=w524:variant)
            n276 = Bundle By Name(cluster=T26 {"Cmd"="Move Focus", "Parameters"=variant} ("element"), "Parameters"=w524) -> (w523:T26)
            n277 = Enqueue Element(queue=w526, element=w523) -> (error out=w519:errorcluster)  [unwired: 2 in, 2 out]
            n278 = call "CC System Message.vi"("Message"="Script commanding telescope to move." ("format string")) -> ()  [unwired: 10 in, 1 out]
            n279 = call "Stall Data Flow.vim"("value in"=w519, "milliseconds to wait"=u32 2000) -> ()  [unwired: 2 out]
            n280 = Bundle By Name(cluster=w520, "Script State"="script Wait for Telescope Move") -> (w521:T24)
          }
          frame "script Telescope Home" {
            # "give telescope time to start\nmoving."
            n281 = Unbundle By Name(w533) -> ("Run Script"=w542:T4[], "step"=w541:i32, "Cmd Qs.Telescope Q"=w539:T2)
            n282 = Index Array(array=w542, index=w541) -> (element=w540:T4)
            n283 = Unbundle By Name(w540) -> ("Data"=w537:variant)
            n284 = Bundle By Name(cluster=T26 {"Cmd"="Home Focus", "Parameters"=variant} ("element"), "Parameters"=w537) -> (w536:T26)
            n285 = call "CC System Message.vi"("Message"="Script commanding telescope to home the focus." ("format string")) -> ()  [unwired: 10 in, 1 out]
            n286 = Enqueue Element(queue=w539, element=w536) -> (error out=w532:errorcluster)  [unwired: 2 in, 2 out]
            n287 = call "Stall Data Flow.vim"("value in"=w532, "milliseconds to wait"=u32 2000) -> ()  [unwired: 2 out]
            n288 = Bundle By Name(cluster=w533, "Script State"="script Wait for Telescope Move") -> (w534:T24)
          }
          frame "script Telescope RA DEC" {
            (unwired) CC_enum_Script_Action."Telescope RA DEC" ("Action")
            # "give telescope time to start\nmoving."
            n289 = Unbundle By Name(w552) -> ("Run Script"=w560:T4[], "step"=w559:i32, "Cmd Qs.Telescope Q"=w557:T2)
            n290 = Index Array(array=w560, index=w559) -> (element=w558:T4)
            n291 = Unbundle By Name(w558) -> ("Data"=w549:variant)
            n292 = Variant To Data(type=T10 {"RA"=0.0, "DEC"=0.0} ("RA and DEC"), Variant=w549) -> (data=w547:T10)  [unwired: 1 in, 1 out]
            n293 = Bundle By Name(cluster=T26 {"Cmd"="Move", "Parameters"=variant} ("element"), "Parameters"=w549) -> (w555:T26)
            n294 = call "CC Convert RA and DEC to HHMMSS.vi"("RA and DEC"=w547) -> ("DEC String"=w545:string, "RA String"=w544:string)  [unwired: 7 in, 2 out]
            n295 = Enqueue Element(queue=w557, element=w555) -> (error out=w551:errorcluster)  [unwired: 2 in, 2 out]
            n296 = Format Into String(format string="Script commanding telescope to move to RA %s, DEC %s.", w544, w545) -> (resulting string=w543:string)  [unwired: 2 in, 1 out]
            n297 = call "CC System Message.vi"("Message"=w543) -> ()  [unwired: 10 in, 1 out]
            n298 = call "Stall Data Flow.vim"("value in"=w551, "milliseconds to wait"=u32 2000) -> ()  [unwired: 2 out]
            n299 = Bundle By Name(cluster=w552, "Script State"="script Wait for Telescope Move") -> (w553:T24)
          }
          frame "script Wait for Telescope Move" {
            n300 = call "CC Log Object.vi"("Action"=CC_enum_Current_Values_Action."Get Current Values") -> ("HK Channel out"=w567:refnum<class "HK Table.lvclass">)  [unwired: 8 in, 2 out]
            n301 = for {
              tunnel: w567 -> [w575]
              tunnel: string[] ["Telescope RA", "Telescope DEC", "Telescope Moving?", "Telescope Status"] -> [w574] mode=indexing
              tunnel: [w573] -> w565 mode=indexing
              n302 = call-dynamic "HK Read Value.vi"("Channel Name"=w574, "HK Channel in"=w575) -> ("Value"=w573:dbl)  [unwired: 4 in, 5 out]
            }
            n303 = Index Array(array=w565) -> (element #3=w564:dbl)  [unwired: 4 in, 3 out]
            n304 = Equal To 0?(x=w564) -> (x = 0?=w563:bool)
            n305 = case shown="False" w563 {
              tunnel: w561 -> [w571 w572]
              tunnel: [w569 w572] -> w562
              frame False {
                n306 = Bundle By Name(cluster=w571, "Script State"="Next Step") -> (w569:T24)
              }
              frame True {
              }
            }
          }
          frame "Ask User", "script Ask User" {
            n307 = Unbundle By Name(w576) -> ("Parameters"=w579:variant)
            n308 = Variant To Data(type="", Variant=w579) -> (data=w582:string, error out=w581:errorcluster)  [unwired: 1 in]
            n309 = case shown="No Error" w581 {
              tunnel: ["User Notification" ("Message") w585] -> w580
              tunnel: w579 -> [_ w587]
              frame No Error {
              }
              frame Error {
                n310 = call <vilib>:"Get Type Information.vi"("variant"=w587) -> ("name"=w586:string)  [unwired: 6 in, 4 out]
                n311 = Format Into String(format string="Software System Error in scripting. Ask User state parameter should be string but was not. Variant contents: %s", w586) -> (resulting string=w585:string)  [unwired: 2 in, 1 out]
              }
            }
            n312 = One Button Dialog(message=w582) -> ()  [unwired: 1 in, 1 out]
            n313 = Bundle By Name(cluster=w576, "Script State"="next step") -> (w577:T24)
            n314 = call "CC System Message.vi"("Message"=w580) -> ()  [unwired: 10 in, 1 out]
          }
          frame "next step" {
            n315 = Unbundle By Name(w592) -> ("step"=w596:i32, "Run Script"=w595:T4[], "paused"=w589:bool)
            n316 = Increment(x=w596) -> (x+1=w591:i32)
            n317 = Array Size(array=w595) -> (size(s)=w594:i32)
            n318 = Greater Or Equal?(x=w591, y=w594) -> (x >= y?=w593:bool)
            n319 = case shown="False" w593 {
              tunnel: w592 -> [w600 w606]
              tunnel: w591 -> [w599 _]
              tunnel: [w598 w607] -> w590
              tunnel: w589 -> [w597 _]
              frame False {
                n320 = case shown="False" w597 {
                  tunnel: w600 -> [w604 w605]
                  tunnel: w599 -> [w603 _]
                  tunnel: [w602 w605] -> w598
                  frame False {
                    n321 = Bundle By Name(cluster=w604, "step"=w603, "Script State"="execute step" ("event data")) -> (w602:T24)
                  }
                  frame True {
                  }
                }
              }
              frame True {
                n322 = Bundle By Name(cluster=w606, "Script State"="end script" ("event data")) -> (w607:T24)
              }
            }
          }
          frame "end script" {
            w612 = "" ("Step Name")
            n323 = Unbundle By Name(w620) -> ("Script Settings.Script Name"=w623:string, "Script Status Q"=w618:refnum<queue>, "Data Q"=w609:refnum<queue>)
            n324 = Get Date/Time In Seconds() -> (seconds since 1Jan1904=w611:timestamp)
            n325 = Format Into String(format string="Script %s finished", w623) -> (resulting string=w624:string)  [unwired: 2 in, 1 out]
            n326 = call "CC Script Send Script End Status.vi"("Data Q"=w609) -> ()  [unwired: 10 in, 1 out]
            n327 = Bundle By Name(cluster=T30 {"Time"=timestamp(0 s since 1904-01-01), "Running"=FALSE, "Step"=0, "Script Name"="", "Step Name"=""}, "Running"=FALSE, "Step"=0, "Step Name"=w612, "Script Name"=w612, "Time"=w611) -> (w610:T30)
            n328 = call "CC System Message.vi"("Message"=w624) -> ()  [unwired: 10 in, 1 out]
            n329 = Bundle By Name(cluster=w620, "Script Running"=FALSE, "Script State"="idle") -> (w621:T24)
            n330 = Bundle By Name(cluster=T28 {"Msg"="Status", "Data"=variant} ("element"), "Data"=w610) -> (w616:T28)
            n331 = Enqueue Element(queue=w618, element=w616) -> ()  [unwired: 2 in, 3 out]
          }
          frame "abort script" {
            n332 = Unbundle By Name(w628) -> ("Script Settings.Script Name"=w630:string, "Script Running"=w627:bool)
            n333 = case shown="False" w627 {
              tunnel: w630 -> [_ w637]
              tunnel: [w632 w636] -> w629
              tunnel: w628 -> [w632 w635]
              tunnel: ["Script Abort received but script not running" w633] -> w626
              frame False {
              }
              frame True {
                n334 = Format Into String(format string="Script %s aborted.", w637) -> (resulting string=w633:string)  [unwired: 2 in, 1 out]
                n335 = Bundle By Name(cluster=w635, "Script State"="end script") -> (w636:T24)
              }
            }
            n336 = call "CC System Message.vi"("Message"=w626) -> ()  [unwired: 10 in, 1 out]
          }
          frame "script error" {
            n337 = Unbundle By Name(w639) -> ("Data Q"=w642:refnum<queue>)
            n338 = call "CC Script Set Status Value.vi"("Value"=2.0, "Ch Name"="Script State", "Data Q"=w642) -> ()  [unwired: 8 in, 1 out]
            n339 = Bundle By Name(cluster=w639, "Script State"="abort script") -> (w643:T24)
          }
          frame "Shutdown" {
            n340 = Unbundle By Name(w647) -> ("Script Settings"=w646:T3)
            n341 = call "Rd Wr Script Defaults.vi"("Write? (F:Read)"=TRUE, "Script Settings"=w646) -> ()  [unwired: 8 in, 2 out]
          }
        }
      }
      event "Script Path": Value Change {
        n342 = event-data() -> ()  [unwired: 1 in, 6 out]
        n343 = Unbundle By Name(w654) -> ("state"=w653:refnum<user-event>)
        n344 = Generate User Event(user event=w653, event data cluster="init" ("event data")) -> ()  [unwired: 2 in, 2 out]
        n345 = Bundle By Name(cluster=w654, "Script Settings.Script Path"="Script Path") -> (w651:T24)
        n346 = Unbundle By Name(w651) -> ("Script Settings"=w650:T3)
        n347 = call "Rd Wr Script Defaults.vi"("Write? (F:Read)"=TRUE, "Script Settings"=w650) -> ()  [unwired: 8 in, 2 out]
      }
      event "Script": Shortcut Menu Activation? {
        n348 = event-data() -> ("CtlRef"=w664:refnum<vi>, "MenuRef"=w662:refnum<k9>, "Coords"=w663:T38)  [unwired: 1 in, 1 out]
        n349 = Unbundle By Name(w657) -> ("Script Settings.Script Path"=w656:path)
        n350 = invoke class="MCListbox (strict)" method="Point To Row Column"(reference=w664, "Point"=w663) -> ()  [unwired: 5 in, 7 out]
        n351 = call "CC Rd Wr Script.vi"("Script Path"=w656, "Action"=CC_Rd_Wr_Script_Action."List") -> ("Script List"=w659:string[])  [unwired: 4 in, 5 out]
        n352 = for {
          tunnel: w659 -> [w667] mode=indexing
          tunnel: [w666] -> w658 mode=indexing
          n353 = Format Into String(format string="Insert|%s", w667) -> (resulting string=w666:string)  [unwired: 2 in, 1 out]
        }
        n354 = Insert Menu Items(5:"Insert" ("menu tag"), 7:w658, 8:w659, 9:w662) -> ()  [unwired: 2 in, 3 out]
        n355 = event-data("Discard?"=FALSE) -> ()  [unwired: 1 in, 1 out]
      }
      event "Script": Shortcut Menu Selection (User) {
        n356 = event-data() -> ("ItemTag"=w676:string, "CtlRef"=w681:refnum<vi>, "Coords"=w680:T38)  [unwired: 1 in, 5 out]
        n357 = Unbundle By Name(w672) -> ("state"=w670:refnum<user-event>, "Script"=w677:T4[], "Script Settings.Script Path"=w669:path)
        n358 = invoke class="MCListbox (strict)" method="Point To Row Column"(reference=w681, "Point"=w680) -> ("CellPosition"=w679:T39)  [unwired: 5 in, 6 out]
        n359 = Match Pattern(string=w676, regular expression="|") -> (before substring=w674:string, after substring=w673:string)  [unwired: 1 in, 2 out]
        n360 = Unbundle By Name(w679) -> ("Row"=w678:i32)
        n361 = case shown="\"Insert\"" w674 {
          tunnel: w678 -> [_ w685 w687 w706]
          tunnel: w677 -> [_ w686 _ w707]
          tunnel: w673 -> [_ _ _ w710]
          tunnel: w672 -> [w682 w683 w688 w701]
          tunnel: [w682 w683 w692 w699] -> w671
          tunnel: w670 -> [_ _ _ w698]
          tunnel: w669 -> [_ _ _ w695]
          frame "False", Default {
          }
          frame "Execute Step" {
            n362 = Index Array(array=w686, index=w685) -> (element=w684:T4)
            n363 = call "CC Script Execute Step.vi"("Script Step"=w684) -> ()  [unwired: 10 in, 1 out]
          }
          frame "Continue From This Step" {
            n364 = Unbundle By Name(w688) -> ("Script Settings.Script Name"=w690:string)
            n365 = Bundle By Name(cluster=w688, "step"=w687, "Script Running"=TRUE, "Script State"="execute step" ("event data")) -> (w692:T24)
            n366 = Format Into String(format string="Continuing Script \"%s\" from step %d" ("Message"), w690, w687) -> (resulting string=w689:string)  [unwired: 2 in, 1 out]
            n367 = call "CC System Message.vi"("Message"=w689) -> ()  [unwired: 10 in, 1 out]
          }
          frame "Insert" {
            n368 = Bundle By Name(cluster=T29 {"Name"="", "Script"=[]} ("Script"), "Name"=w710) -> (w709:T29)
            n369 = Increment(x=w706) -> (x+1=w696:i32)
            n370 = Generate User Event(user event=w698, event data cluster="show script" ("event data")) -> ()  [unwired: 2 in, 2 out]
            n371 = Split 1D Array(array=w707, index=w696) -> (first subarray=w703:T4[], second subarray=w704:T4[])
            n372 = call "CC Rd Wr Script.vi"("Script Path"=w695, "Action"=CC_Rd_Wr_Script_Action."Read", "Script"=w709) -> ("Script"=w705:T29)  [unwired: 3 in, 5 out]
            n373 = Unbundle By Name(w705) -> ("Script"=w702:T4[])
            n374 = Build Array (concatenate)(w703, w702, w704) -> (w700:T4[])
            n375 = Bundle By Name(cluster=w701, "Script"=w700) -> (w699:T24)
          }
        }
      }
      event "Script": Value Change {
        n376 = event-data() -> ("NewVal"=w716:string)  [unwired: 1 in]
        n377 = Unbundle By Name(w714) -> ("state"=w713:refnum<user-event>)
        n378 = Generate User Event(user event=w713, event data cluster="load script" ("event data")) -> ()  [unwired: 2 in, 2 out]
        n379 = Bundle By Name(cluster=w714, "Script Settings.Script Name"=w716) -> (w715:T24)
      }
      event "Edit Script", "New Script": Value Change {
        n380 = event-data() -> ()  [unwired: 1 in, 6 out]
        n381 = Unbundle By Name(w719) -> ("script edit ref"=w718:refnum<vi>)
        n382 = property class="VI Interface Type 0"(reference=w718) -> ("FP.State"=w717:T40)  [unwired: 1 in, 2 out]
        n383 = Select(t="", s="New Script", f="Script") -> (s? t:f=w721:string)
        n384 = case shown="\"Invalid\", Default" w717 {
          tunnel: w721 -> [w729 _]
          tunnel: [w728 w736] -> w720
          tunnel: w719 -> [w727 w736]
          tunnel: w718 -> [_ w738]
          frame "Invalid", Default {
            n385 = vi-ref "CC Create Script.vi"() -> (w734:refnum<vi>)
            n386 = property class="VI (strict)"(reference=w734) -> (error out=w735:errorcluster, "Path"=w733:path)  [unwired: 1 in, 1 out]
            n387 = Open VI Reference(type specifier VI Refnum (for type only)=w734, vi path=w733, options=128, error in (no error)=w735) -> (vi reference=w732:refnum<vi>, error out=w730:errorcluster)  [unwired: 2 in]
            n388 = call-by-ref "Start Asynchronous Call"(reference=w732, error in=w730, "script name in"=w729) -> (reference out=w726:refnum<vi>)  [unwired: 10 in, 2 out]
            n389 = Bundle By Name(cluster=w727, "script edit ref"=w726) -> (w728:T24)
            n390 = invoke class="VI (strict)" method="FP.Open"(reference=w726, "Activate"=TRUE ("Activate?")) -> ()  [unwired: 3 in, 5 out]
          }
          frame "Standard" {
            n391 = property class="VI Interface Type 0"(reference=w738, "Front Panel.IsFrontmost"=TRUE ("Front Panel Window:Is Frontmost")) -> ()  [unwired: 1 in, 2 out]
          }
        }
      }
      event "Run Script": Value Change {
        n392 = event-data() -> ()  [unwired: 1 in, 6 out]
        n393 = Unbundle By Name(w741) -> ("state"=w740:refnum<user-event>)
        n394 = Generate User Event(user event=w740, event data cluster="start script" ("event data")) -> ()  [unwired: 2 in, 2 out]
      }
      event "Stop Script": Value Change {
        n395 = event-data() -> ()  [unwired: 1 in, 6 out]
        n396 = Unbundle By Name(w744) -> ("state"=w743:refnum<user-event>)
        n397 = Generate User Event(user event=w743, event data cluster="abort script" ("event data")) -> ()  [unwired: 2 in, 2 out]
      }
      event "Close": Value Change {
        n398 = event-data() -> ()  [unwired: 1 in, 2 out]
        n399 = Unbundle By Name(w747) -> ("state"=w746:refnum<user-event>)
        n400 = Generate User Event(user event=w746, event data cluster="shutdown" ("event data")) -> ()  [unwired: 2 in, 2 out]
      }
    }
  }
